vi "FormatMethodCall.vi"(1 "method":string, 2 "parameters":string[](array[string]), 3 "object":string) -> (0 "python object":string)   [LabVIEW 2014, in "Raspberry Pi Compatible Compiler for LabVIEW.lvlib" / "Python Functions.lvlib"]
uses:
  Python Functions.lvlib
  ListTypesTD.ctl
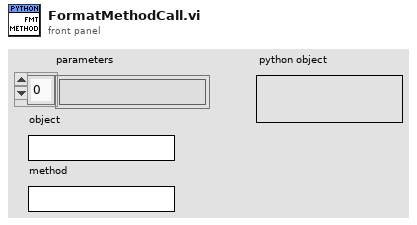
[diagram p1: front panel]
types:
  T1 = typedef "Raspberry Pi Compatible Compiler for LabVIEW.lvlib/Python Functions.lvlib/ListTypesTD.ctl" = enum16{"list", "tuple", "parameter list", "output list", "return values"}
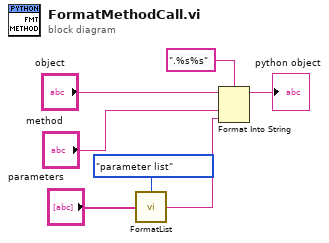
[diagram p0: block diagram]
diagram:
  n1 = call "FormatList.vi"("values"="parameters", "type"=ListTypesTD."parameter list") -> ("python object"=w2:string)
  n2 = Format Into String(format string=".%s%s", initial string="object", "method", w2) -> (resulting string=→"python object":string)  [unwired: 1 in, 1 out]
